vi "Zero-Order Hold (DBL).vi"(2 "initialize":bool, 3 "hold time in cycles":i32, 5 "input point":dbl format="%.2f") -> (1 "output point":dbl format="%.2f")   [LabVIEW 2017, in "NI_AdvCtrl_discrete linear.lvlib"]
doc: "LabVIEW no longer supports this VI. You can obtain similar functionality by installing the LabVIEW Simulation Module.\n\nHolds the signal for a definite period of time. In other words, the prediction of the signal is based only on the current input point."
uses:
  <vilib>/addons/control/advanced/NI_AdvCtrl_discrete linear.lvlib
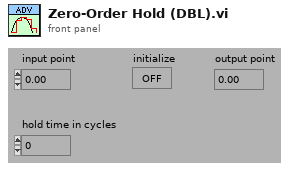
[diagram p1: front panel]
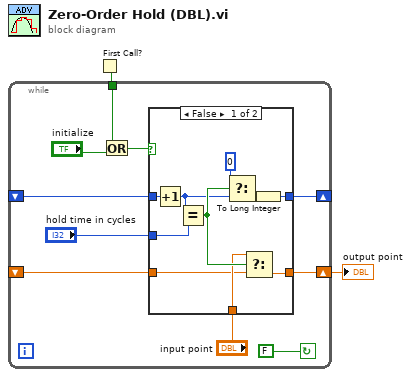
[diagram p0: block diagram]
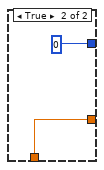
[diagram p2: hidden frame]
diagram:
  n1 = First Call?() -> (First Call?: T/F=w1:bool)
  n2 = while {
    tunnel: w1 -> [w4]
    shift-left: _ -> [w10]
    shift-right: [w11] -> _
    shift-left: _ -> [w9]
    shift-right: [w12] -> w2
    stop <- FALSE continue-if-true
    n3 = Or(x=w4, y="initialize") -> (x .or. y?=w3:bool)
    n4 = case shown="False" w3 {
      tunnel: [w13 0] -> w11
      tunnel: [w14 w23] -> w12
      tunnel: w10 -> [w22 _]
      tunnel: w9 -> [w15 _]
      tunnel: "input point" -> [w16 w23]
      tunnel: "hold time in cycles" -> [w21 _]
      frame False {
        n5 = Increment(x=w22) -> (x+1=w19:i32)
        n6 = Equal?(x=w19, y=w21) -> (x = y?=w20:bool)
        n7 = Select(t=0, s=w20, f=w19) -> (s? t:f=w17:i32)
        n8 = Select(t=w16, s=w20, f=w15) -> (s? t:f=w14:dbl)
        n9 = To Long Integer(number=w17) -> (32bit integer=w13:i32)
      }
      frame True {
      }
    }
  }
  "output point" <- w2
